vi "Set Solonoid.vi"(8 "error in (no error)":errorcluster, 10 "State":bool, 11 "Feeder Actor.lvlib:Solenoid.lvclass":refnum<class "Solenoid.lvclass">) -> (0 "error out":errorcluster, 3 "Feeder Actor.lvlib:Solenoid.lvclass 2":refnum<class "Solenoid.lvclass">)   [LabVIEW 2018, in "Feeder Actor.lvlib" / "Solenoid.lvclass"]
uses:
  Solenoid.lvclass
  Solenoid.lvclass/Solenoid.ctl
  <vilib>/DAQmx/write.llb/DAQmx Write (Digital Bool 1Line 1Point).vi
  <vilib>/DAQmx/miscellaneous.llb/DAQmx Fill In Error Info.vi
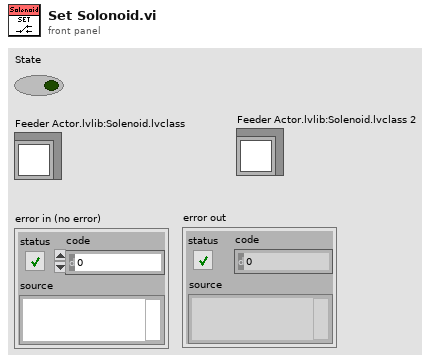
[diagram p1: front panel]
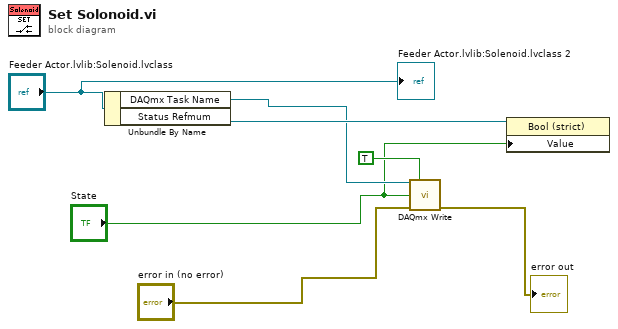
[diagram p0: block diagram]
diagram:
  n1 = Unbundle By Name("Feeder Actor.lvlib:Solenoid.lvclass") -> ("DAQmx Task Name"=w5:refnum<k21>, "Status Refmum"=w7:refnum<vi>)
  n2 = call-poly <vilib>:"DAQmx Write.vi"("task/channels in"=w5, "auto start"=TRUE, "data"="State", "error in"="error in (no error)") -> ("error out"=→"error out":errorcluster)  [unwired: 9 in, 2 out]
  n3 = property class="Bool (strict)"(reference=w7, "Value"="State") -> ()  [unwired: 1 in, 2 out]
  "Feeder Actor.lvlib:Solenoid.lvclass 2" <- "Feeder Actor.lvlib:Solenoid.lvclass"
